vi "TC-01-(Acquire)AcquireFromDevice.vi"(8 "error in (no error)":errorcluster, 11 "NI-TC-01 in":refnum<class "NI-TC-01.lvclass">) -> (0 "error out":errorcluster, 3 "NI-TC-01 out":refnum<class "NI-TC-01.lvclass">)   [LabVIEW 2020, in "NI-TC-01.lvclass"]
uses:
  NI-TC-01.lvclass
  NI-TC-01.lvclass/NI-TC-01.ctl
  <vilib>/DAQmx/read.llb/DAQmx Read (Analog DBL 1Chan 1Samp).vi
  <vilib>/DAQmx/miscellaneous.llb/DAQmx Fill In Error Info.vi
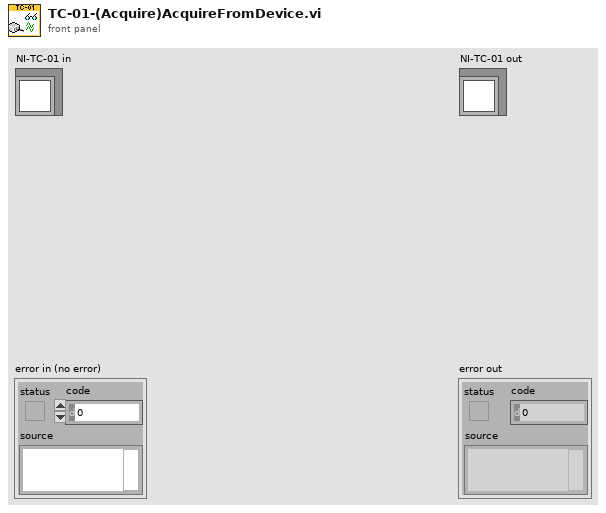
[diagram p1: front panel]
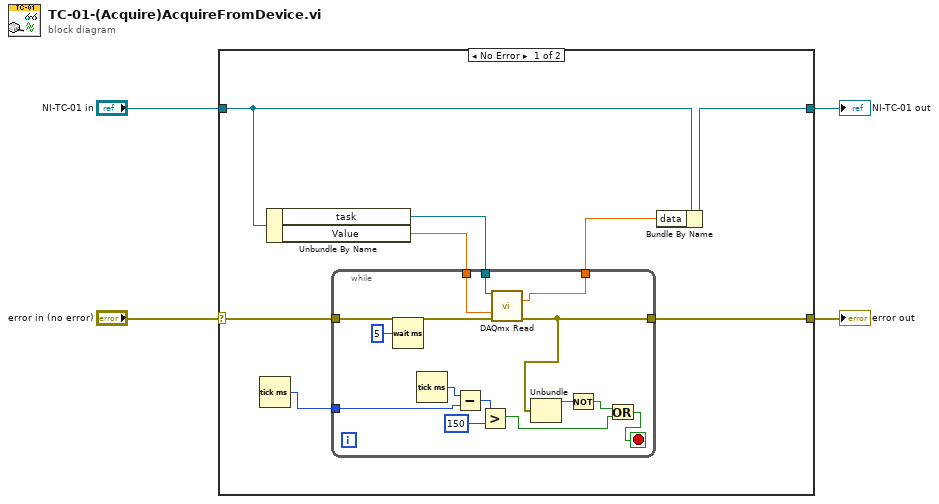
[diagram p0: block diagram]
diagram:
  n1 = case shown="No Error" "error in (no error)" {
    selector: "error in (no error)" -> [w10 w28]
    tunnel: [w9 w28] -> w3
    tunnel: [w7 w27] -> w1
    tunnel: "NI-TC-01 in" -> [w8 w27]
    frame No Error {
      n2 = Tick Count (ms)() -> (millisecond timer value=w5:u32)
      n3 = Unbundle By Name(w8) -> ("task"=w12:refnum<k21>, "Value"=w11:dbl)
      n4 = while {
        tunnel: w12 -> [w26]
        tunnel: w11 -> [w25]
        tunnel: w10 -> [w24]
        tunnel: [w22] -> w9
        tunnel: [w23] -> w6
        tunnel: w5 -> [w19]
        stop <- w13 stop-if-true
        n5 = Wait (ms)(milliseconds to wait=u32 5) -> ()  [unwired: 1 out]
        n6 = Tick Count (ms)() -> (millisecond timer value=w20:u32)
        n7 = Subtract(x=w20, y=w19) -> (x-y=w18:u32)
        n8 = Greater?(x=w18, y=u32 150) -> (0:w14:bool)
        n9 = call-poly <vilib>:"DAQmx Read.vi"("task/channels in"=w26, "timeout"=w25, "error in"=w24) -> ("data"=w23:dbl, "error out"=w22:errorcluster)  [unwired: 10 in, 1 out]
        n10 = Unbundle(w22) -> ("status"=w21:bool)  [unwired: 2 out]
        n11 = Not(x=w21) -> (.not. x?=w15:bool)
        n12 = Or(x=w15, y=w14) -> (x .or. y?=w13:bool)
      }
      n13 = Bundle By Name(cluster=w8, "data"=w6) -> (w7:refnum<class "NI-TC-01.lvclass">)
    }
    frame Error {
    }
  }
  "error out" <- w3
  "NI-TC-01 out" <- w1
